vi "PH_Timing.configure PU Channel.vi"(0 "i ref in":refnum<vi>, 1 "GateGen Instance":string="N/A", 3 "Channel":i32(ring)=1 items=["System (To)", "Channel A", "Channel B", "Channel C", "Channel D", "Channel E", "Channel F", "Channel G", "Channel H"], 4 "Delay":dbl, 5 "error in":errorcluster) -> (14 "i ref out":refnum<vi>, 19 "error out":errorcluster)   [LabVIEW 2014, in "PH_Timing.lvlib"]
doc: "Within this VI a BNC555 Gate and Delay Generator channel is specifically confugred with PU settings."
uses:
  PH_Timing.lvlib
  CS_DigitalIO/BNC555/BNC555.lvlib
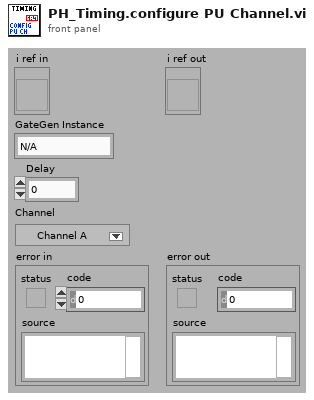
[diagram p1: front panel]
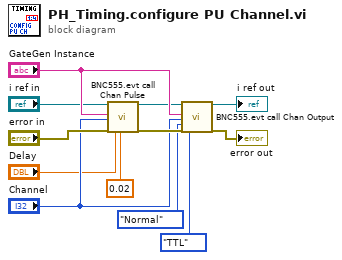
[diagram p0: block diagram]
diagram:
  n1 = call "BNC555.evt call Chan Pulse.vi"("i ref in"="i ref in", "Generator Instance"="GateGen Instance", "Channel"="Channel", "error in (no error)"="error in", "Delay"="Delay", "Width"=0.02 ("Pulse Width [s] (4e-9s)")) -> ("i ref out"=w6:refnum<vi>, "error out"=w7:errorcluster)  [unwired: 12 in]
  n2 = call "BNC555.evt call Chan Output.vi"("i ref in"=w6, "Generator Instance"="GateGen Instance", "Channel"="Channel", "Polarity (Normal)"=enum16{"Normal", "Complement", "Inverted"}."Normal", "error in (no error)"=w7, "Level (TTL)"=enum16{"TTL", "Adjustable", "35 Volt"}."TTL") -> ("i ref out"=→"i ref out":refnum<vi>, "error out"=→"error out":errorcluster)  [unwired: 12 in]
